vi "Print Plot.vi"(0 "File:":string, 1 "X-Axis Label":string="Field (tesla)", 2 "Data Plot":cluster{dbl[], dbl[]}[](graph)) -> ()   [LabVIEW 2021]
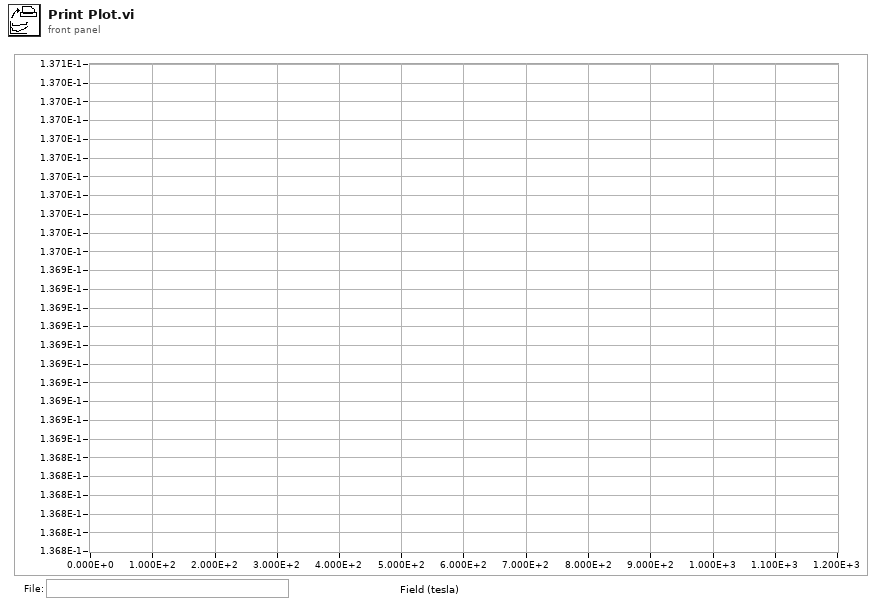
[diagram p1: front panel]
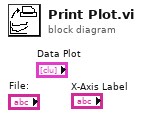
[diagram p0: block diagram]
diagram:
